vi "File.Copy, Overwrite if Exists.vi"(8 "error in":errorcluster, 10 "Target Path":path, 11 "Source Path":path) -> (0 "error out":errorcluster, 3 "Target Out":path)   [LabVIEW 2024]
uses:
  Errors/Error.Error Code List.ctl
  Errors.lvlib
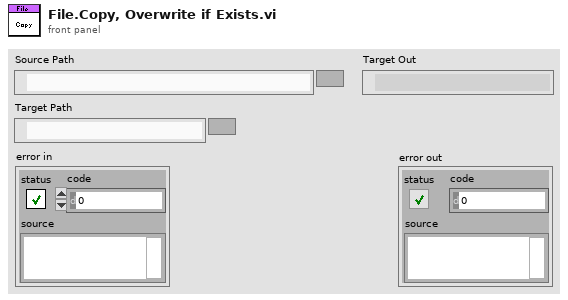
[diagram p1: front panel]
types:
  T1 = typedef "EQMF.lvlib/Errors.lvlib/Error.Error Code List.ctl" = i32
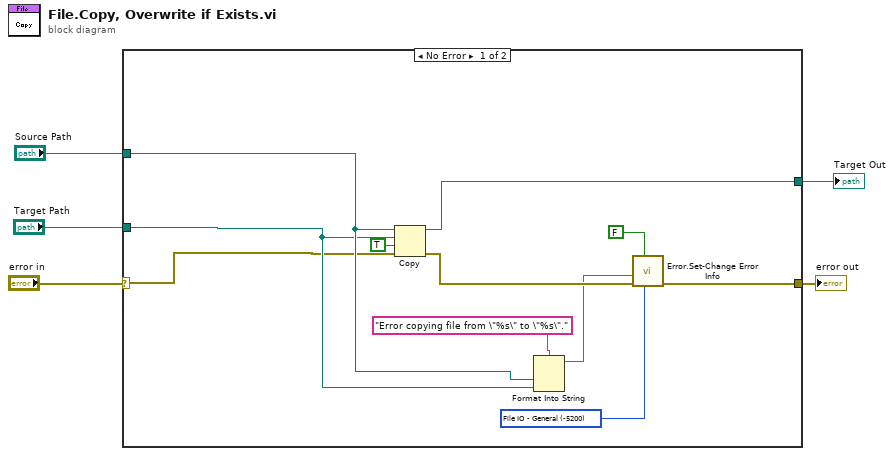
[diagram p0: block diagram]
diagram:
  n1 = case shown="No Error" "error in" {
    selector: "error in" -> [w6 w18]
    tunnel: "Target Path" -> [w7 w17]
    tunnel: [w14 w18] -> w4
    tunnel: "Source Path" -> [w12 _]
    tunnel: [w16 w17] -> w1
    frame No Error {
      w10 = T1 -5200 items=["No Error"=0, "Abort"=-2, "Misc"=-5000, "Fixture Error"=-5100, "File IO - General"=-5200, "FIle IO - Config Error"=-5201, "Instrument - General"=-5300, "Instrument - Serial Com"=-5301, "Instrument - Camera"=-5302, "Instrument - PS"=-5303, "Instrument - Oscilloscope"=-5304, "Instrument - Function Gen"=-5305, "Instrument - Load"=-5306, "Instrument - Meter"=-5307, "Instrument - Power Control"=-5308, "Instrument - Motion"=-5309, "Instrument - RF"=-5310, "System Exe"=-5400, "Image Processing"=-5500, "Communication"=-5600, "Script - Syntax Error"=-6000, "Script - Invalid Name or Param"=-6100, "Script - Timeout"=-6200, "Invalid Data"=-6300, "FW Update Error"=-6500] ("Std Code")
      n2 = Copy(8:w6, 9:TRUE ("overwrite (F)"), 10:w7, 11:w12) -> (0:w15:errorcluster, 3:w16:path)  [unwired: 1 in, 1 out]
      n3 = Format Into String(format string="Error copying file from \"%s\" to \"%s\".", w12, w7) -> (resulting string=w11:string)  [unwired: 2 in, 1 out]
      n4 = call "Error.Set-Change Error Info.vi"("Std Code"=w10, "Append Details"=FALSE, "error in"=w15, "Description"=w11) -> ("error out"=w14:errorcluster)  [unwired: 7 in]
    }
    frame Error {
    }
  }
  "error out" <- w4
  "Target Out" <- w1
